vi "SetTriggerHW.vi"(8 "error in (no error)":errorcluster, 11 "BME_DG_G08 in":refnum<class "BME_DG_G08.lvclass">) -> (0 "error out":errorcluster, 3 "BME_DG_G08 out":refnum<class "BME_DG_G08.lvclass">)   [LabVIEW 2009, in "POLARIS BME DG.lvlib" / "BME_DG_G08.lvclass"]
doc: "VI overwrites and call VI of parent class BME_DG_G05P2. Additional it calls DLL Set_G08_TriggerParameters\n\n\nauthor: Alexander Kessler, Helmholtz-Institut-Jena \nmaintainer: Alexander Kessler: alexander.kessler@uni-jena.de\n\nLast Change:\nLicense Agreement for this software:\n\nCopyright (C)\nHelmholtz-Institut-Jena\nFröbelsteg 3\n07743 Jena\nGermany\n\nContact: alexander.kessler@uni-jena.de\n\nThis program is free software; you can redistribute it and/or modify it under the terms of the GNU General Public License as published by the Free Software Foundation; either version 2 of the license, or (at your option) any later version.\n\nThis program is distributed in the hope that it will be useful, but WITHOUT ANY WARRANTY; without even the implied warranty of MERCHANTABILITY or FITNESS FOR A PARTICULAR PURPOSE. See the GNU General License for more details (http://www.gnu.org)."
uses:
  BME_DG_G08.lvclass
  LV-BME Interface/BME_DG_V2TriggerSettings.ctl
  LV-BME Interface/MSBusSignals.ctl
  LV-BME Interface/SG08_Settings.ctl
  BME_DG_G05P2/BME_DG_G05P2.lvclass
  BME_DG_G08.lvclass/BME_DG_G08.ctl
  POLARIS BME DG.lvlib
panel:
  in  "BME_SG08_Settings":T4={"V2 Trigger Settings"={"Trigger on MS Bus"=24, "Force Trigger (µs)"=0.0, "Gate Type"=TRUE, "Synchronize Gate"=FALSE}, "SG08_Settings"={"Gate Terminate"=TRUE, "Gate Level"=1.0, "Gate Delay (µs)"=0.0, "StepBackTime (µs)"=0.0, "Burst Counter"=0, "Trigger Divider"=1, "Trigger Multiplier"=4}} {"SG08_Settings"."StepBackTime (µs)" min=0.0 format="%.6f"; "SG08_Settings"."Gate Delay (µs)" format="%.3f"; "SG08_Settings"."Gate Level" min=-2.5 max=2.5 format="%.3g"; "V2 Trigger Settings"."Trigger on MS Bus" format="%04x" items=["Local Primary0x1"=1, "Local Secondary0x2"=2, "Local Force 0x4"=4, "Resynchronize 0x8"=8, "StepBackOnBus 0x10"=16, "StartOnBus 0x20"=32, "InhibitOnBus 0x40"=64, "LoadDataOnBus 0x80"=128]; "V2 Trigger Settings"."Force Trigger (µs)" min=0.0 format="%.6f"}
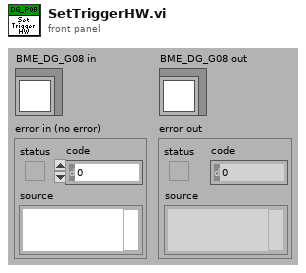
[diagram p1: front panel]
types:
  T1 = typedef "POLARIS BME DG.lvlib/BME_DG_V2TriggerSettings.ctl" = cluster{"Trigger on MS Bus":T2, "Force Trigger (µs)":dbl, "Gate Type":bool, "Synchronize Gate":bool}
  T2 = typedef "POLARIS BME DG.lvlib/MSBusSignals.ctl" = u32
  T3 = typedef "POLARIS BME DG.lvlib/SG08_Settings.ctl" = cluster{"Gate Terminate":bool, "Gate Level":dbl, "Gate Delay (µs)":dbl, "StepBackTime (µs)":dbl, "Burst Counter":u32, "Trigger Divider":u32, "Trigger Multiplier":u32}
  T4 = cluster{"V2 Trigger Settings":T1, "SG08_Settings":T3}
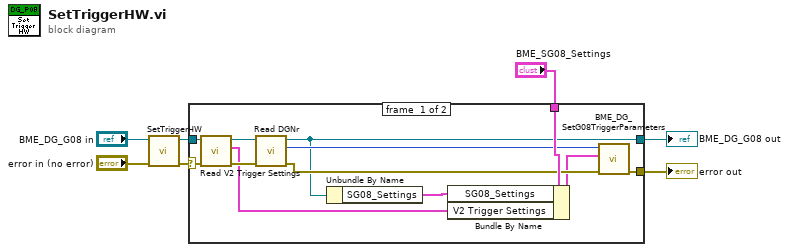
[diagram p0: block diagram]
diagram:
  n1 = call-parent "SetTriggerHW.vi"("error in (no error)"="error in (no error)", "BME_DG_G05 in"="BME_DG_G08 in") -> ("error out"=w3:errorcluster, "BME_DG_G05 out"=w4:refnum<class "BME_DG_G08.lvclass">)  [unwired: 8 in]
  n2 = case shown="No Error" w3 {
    selector: w3 -> [w18 w20]
    tunnel: [w13 w20] -> w7
    tunnel: [w9 w21] -> w6
    tunnel: w4 -> [w15 w21]
    tunnel: "BME_SG08_Settings" -> [w19 _]
    frame #0 {
      n3 = call-dynamic "Read V2 Trigger Settings.vi"("error in (no error)"=w18, "BME_DG_G05 in"=w15) -> ("error out"=w16:errorcluster, "V2 Trigger Settings"=w11:T1, "BME_DG_G05 out"=w17:refnum<class "BME_DG_G08.lvclass">)  [unwired: 7 in]
      n4 = call-dynamic "Read DGNr.vi"("error in (no error)"=w16, "BME_DG_Base in"=w17) -> ("error out"=w14:errorcluster, "DGNr"=w12:i32, "BME_DG_Base out"=w9:refnum<class "BME_DG_G08.lvclass">)  [unwired: 7 in]
      n5 = Unbundle By Name(w9) -> ("SG08_Settings"=w8:T3)
      n6 = Bundle By Name(cluster=w19, "SG08_Settings"=w8, "V2 Trigger Settings"=w11) -> (w10:T4)
      n7 = call "BME_DG_SetG08TriggerParameters.vi"("error in (no error)"=w14, "BME_SG08_Settings"=w10, "DG Number"=w12) -> ("error out"=w13:errorcluster)  [unwired: 8 in]
    }
    frame #1 {
    }
  }
  "BME_DG_G08 out" <- w6
  "error out" <- w7
